vi "Speed test.vi"() -> ()   [LabVIEW 2021]
panel:
  out "FPS":dbl
  out "2D Picture":picture
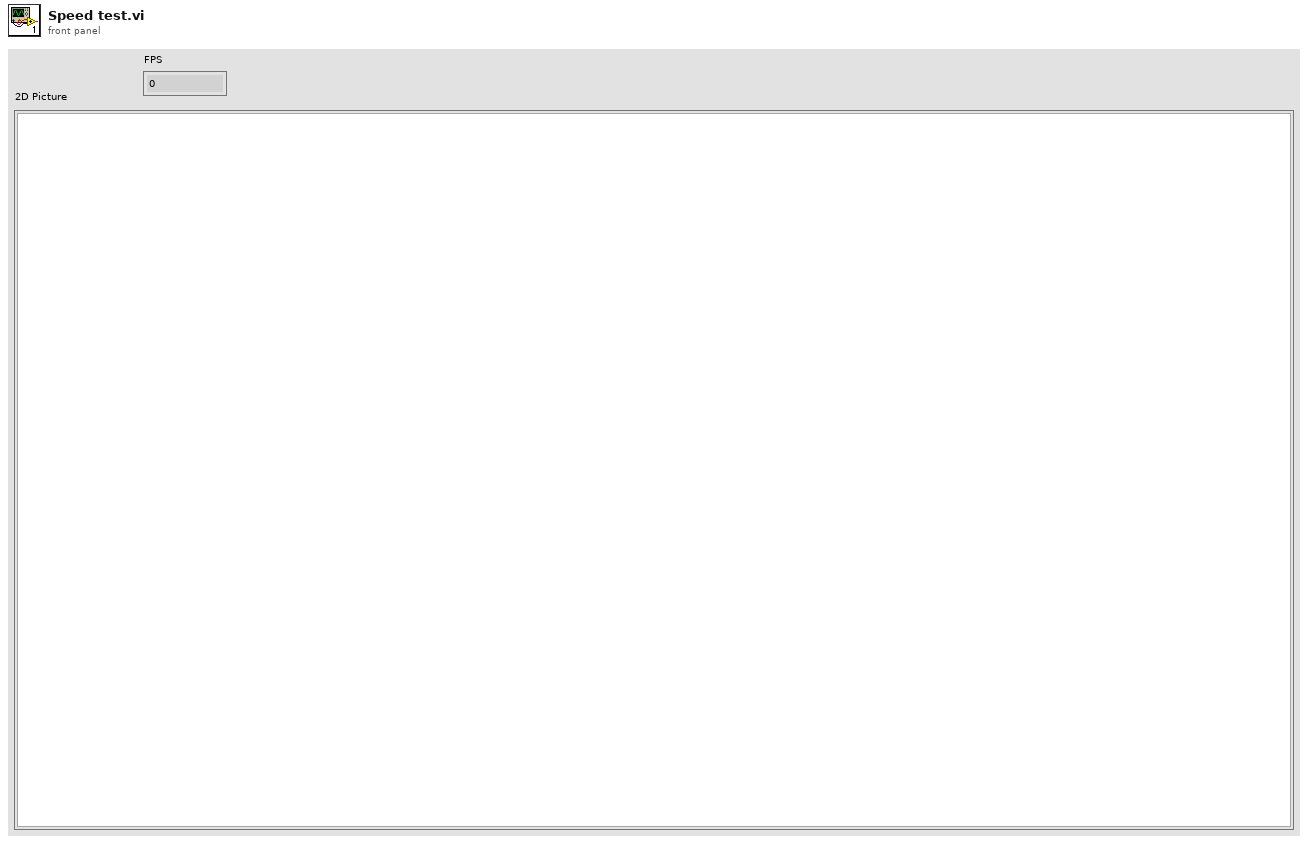
[diagram p1: front panel]
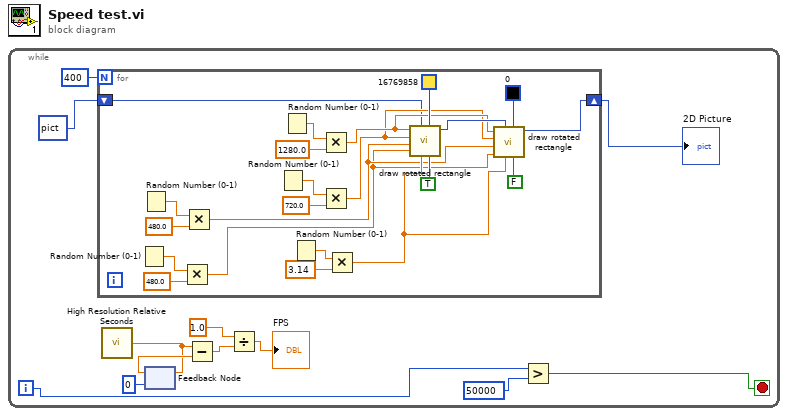
[diagram p0: block diagram]
diagram:
  n1 = while {
    i -> [w6]
    stop <- w4 stop-if-true
    n2 = for {
      N: 400 -> [_]
      shift-right: [w13] -> w2
      shift-left: picture data[5B] ("new picture") -> [w14]
      n3 = Random Number (0-1)() -> (number: 0 to 1=w19:dbl)
      n4 = Random Number (0-1)() -> (number: 0 to 1=w21:dbl)
      n5 = Multiply(x=w19, y=480.0) -> (x*y=w15:dbl)
      n6 = Multiply(x=w21, y=480.0) -> (x*y=w16:dbl)
      n7 = Random Number (0-1)() -> (number: 0 to 1=w23:dbl)
      n8 = Random Number (0-1)() -> (number: 0 to 1=w25:dbl)
      n9 = Random Number (0-1)() -> (number: 0 to 1=w29:dbl)
      n10 = Multiply(x=w25, y=1280.0) -> (x*y=w18:dbl)
      n11 = Multiply(x=w23, y=720.0) -> (x*y=w17:dbl)
      n12 = Multiply(x=w29, y=3.14) -> (x*y=w27:dbl)
      n13 = call "draw rotated rectangle.vi"("fill"=TRUE, "Color Box"=u32 16769858, "angle"=w27, "2D Picture"=w14, "height"=w15, "width"=w16, "y"=w17, "x"=w18) -> ("new picture"=w33:picture)  [unwired: 3 in]
      n14 = call "draw rotated rectangle.vi"("fill"=FALSE, "Color Box"=u32 0, "angle"=w27, "2D Picture"=w33, "height"=w15, "width"=w16, "y"=w17, "x"=w18) -> ("new picture"=w13:picture)  [unwired: 3 in]
    }
    "2D Picture" <- w2
    n15 = call <vilib>:"High Resolution Relative Seconds.vi"() -> ("relative seconds"=w7:dbl)
    n16 = feedback #1(u32 0 ("millisecond timer value")) -> (w8:dbl)
    n17 = feedback-in #1(w7) -> ()
    n18 = Subtract(x=w7, y=w8) -> (x-y=w12:dbl)
    n19 = Divide(x=1.0, y=w12) -> (x/y=→"FPS":dbl)
    n20 = Greater?(x=w6, y=50000) -> (0:w4:bool)
  }
